vi "Manage Data Queue.vi"(8 "error in (no error)":errorcluster, 9 "Add Data (1)":dbl=1.0, 10 "Operation (0: Add Data)":i32(ring) items=["Add Data", "Get Next Data", "Clear Data Queue"], 11 "VISA resource name":refnum<visa-resource-name>) -> (0 "error out":errorcluster, 2 "Result":dbl, 3 "VISA resource name out":refnum<visa-resource-name>)   [LabVIEW 2015, in "Keithley 2600 Series.lvlib"]
doc: "Manages the data queue."
uses:
  Keithley 2600 Series.lvlib
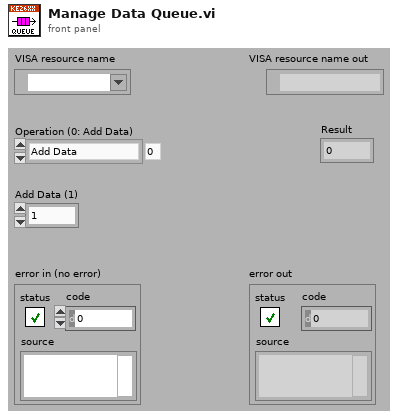
[diagram p1: front panel]
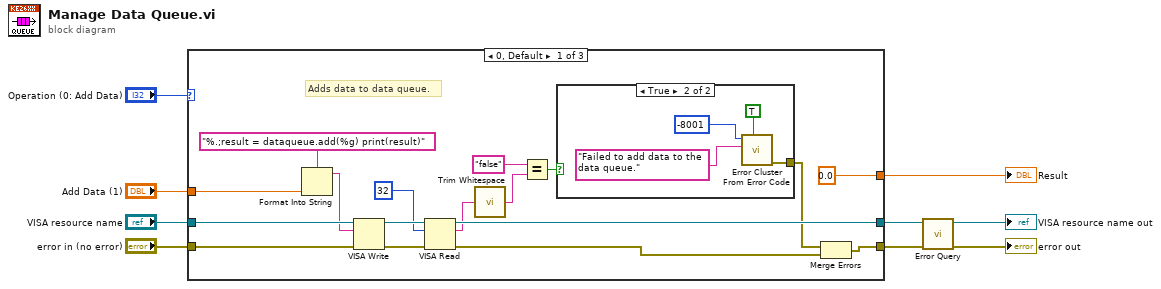
[diagram p0: block diagram]
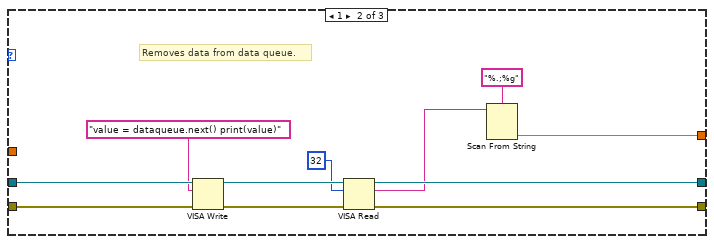
[diagram p3: hidden frame]
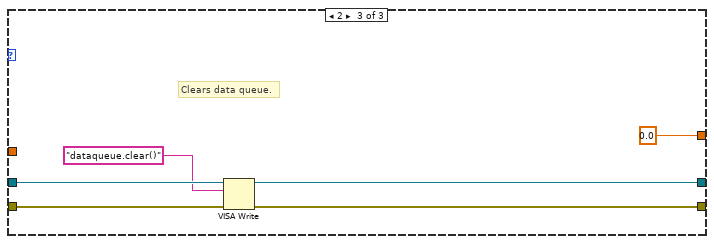
[diagram p4: hidden frame]
diagram:
  n1 = case shown="0, Default" "Operation (0: Add Data)" {
    tunnel: "Add Data (1)" -> [w21 _ _]
    tunnel: "VISA resource name" -> [w26 w39 w47]
    tunnel: "error in (no error)" -> [w25 w38 w46]
    tunnel: [w18 w35 w45] -> w3
    tunnel: [w12 w34 w44] -> w2
    tunnel: [0.0 w31 0.0] -> w1
    frame 0, Default {
      # "Adds data to data queue."
      n2 = Format Into String(format string="%.;result = dataqueue.add(%g) print(result)", w21) -> (resulting string=w20:string)  [unwired: 2 in, 1 out]
      n3 = VISA Write(VISA resource name=w26, write buffer=w20, error in (no error)=w25) -> (VISA resource name out=w24:refnum<visa-resource-name>, error out=w23:errorcluster)  [unwired: 1 out]
      n4 = VISA Read(VISA resource name=w24, byte count=u32 32, error in (no error)=w23) -> (VISA resource name out=w18:refnum<visa-resource-name>, read buffer=w16:string, error out=w10:errorcluster)  [unwired: 1 out]
      n5 = call <vilib>:"Trim Whitespace.vi"("string"=w16) -> ("trimmed string"=w15:string)  [unwired: 1 in]
      n6 = Equal?(x="false", y=w15) -> (x = y?=w14:bool)
      n7 = case shown="True" w14 {
        tunnel: [_ w30] -> w11
        frame False {
        }
        frame True {
          n8 = call <vilib>:"Error Cluster From Error Code.vi"("show call chain? (False)"=TRUE, "error message (\"\")"="Failed to add data to the data queue." ("error message (\"\")"), "error code (0)"=-8001) -> ("error out"=w30:errorcluster)  [unwired: 6 in]
        }
      }
      n9 = Merge Errors(w11, w10) -> (w12:errorcluster)
    }
    frame 1 {
      # "Removes data from data queue."
      n10 = VISA Write(VISA resource name=w39, write buffer="value = dataqueue.next() print(value)", error in (no error)=w38) -> (VISA resource name out=w41:refnum<visa-resource-name>, error out=w40:errorcluster)  [unwired: 1 out]
      n11 = VISA Read(VISA resource name=w41, byte count=u32 32, error in (no error)=w40) -> (VISA resource name out=w35:refnum<visa-resource-name>, read buffer=w33:string, error out=w34:errorcluster)  [unwired: 1 out]
      n12 = Scan From String(format string="%.;%g", input string=w33) -> (output 1=w31:dbl)  [unwired: 3 in, 3 out]
    }
    frame 2 {
      # "Clears data queue."
      n13 = VISA Write(VISA resource name=w47, write buffer="dataqueue.clear()", error in (no error)=w46) -> (VISA resource name out=w45:refnum<visa-resource-name>, error out=w44:errorcluster)  [unwired: 1 out]
    }
  }
  "Result" <- w1
  n14 = call "Error Query.vi"("error in (no error)"=w2, "VISA resource name"=w3) -> ("error out"=→"error out":errorcluster, "VISA resource name out"=→"VISA resource name out":refnum<visa-resource-name>)  [unwired: 6 in, 2 out]
